vi "Matrix_Transpose.vi"(11 "input matrix":T1) -> (3 "output matrix":T1)   [LabVIEW 2019, in "Trajectory_Library.lvlib"]
doc: "Transpose matrix\n \nInputs:\n - input matrix -- The input matrix\n\nOutputs:\n - output matrix -- The transposed matrix"
uses:
  <vilib>/Analysis/Matrix/Datatypes/RealMatrix.ctl
  Trajectory_Library.lvlib
  <vilib>/Analysis/Matrix/NI_Matrix.lvlib
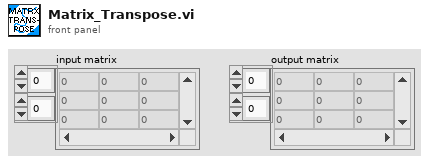
[diagram p1: front panel]
types:
  T1 = typedef "NI_Matrix.lvlib/RealMatrix.ctl" = dbl[][]
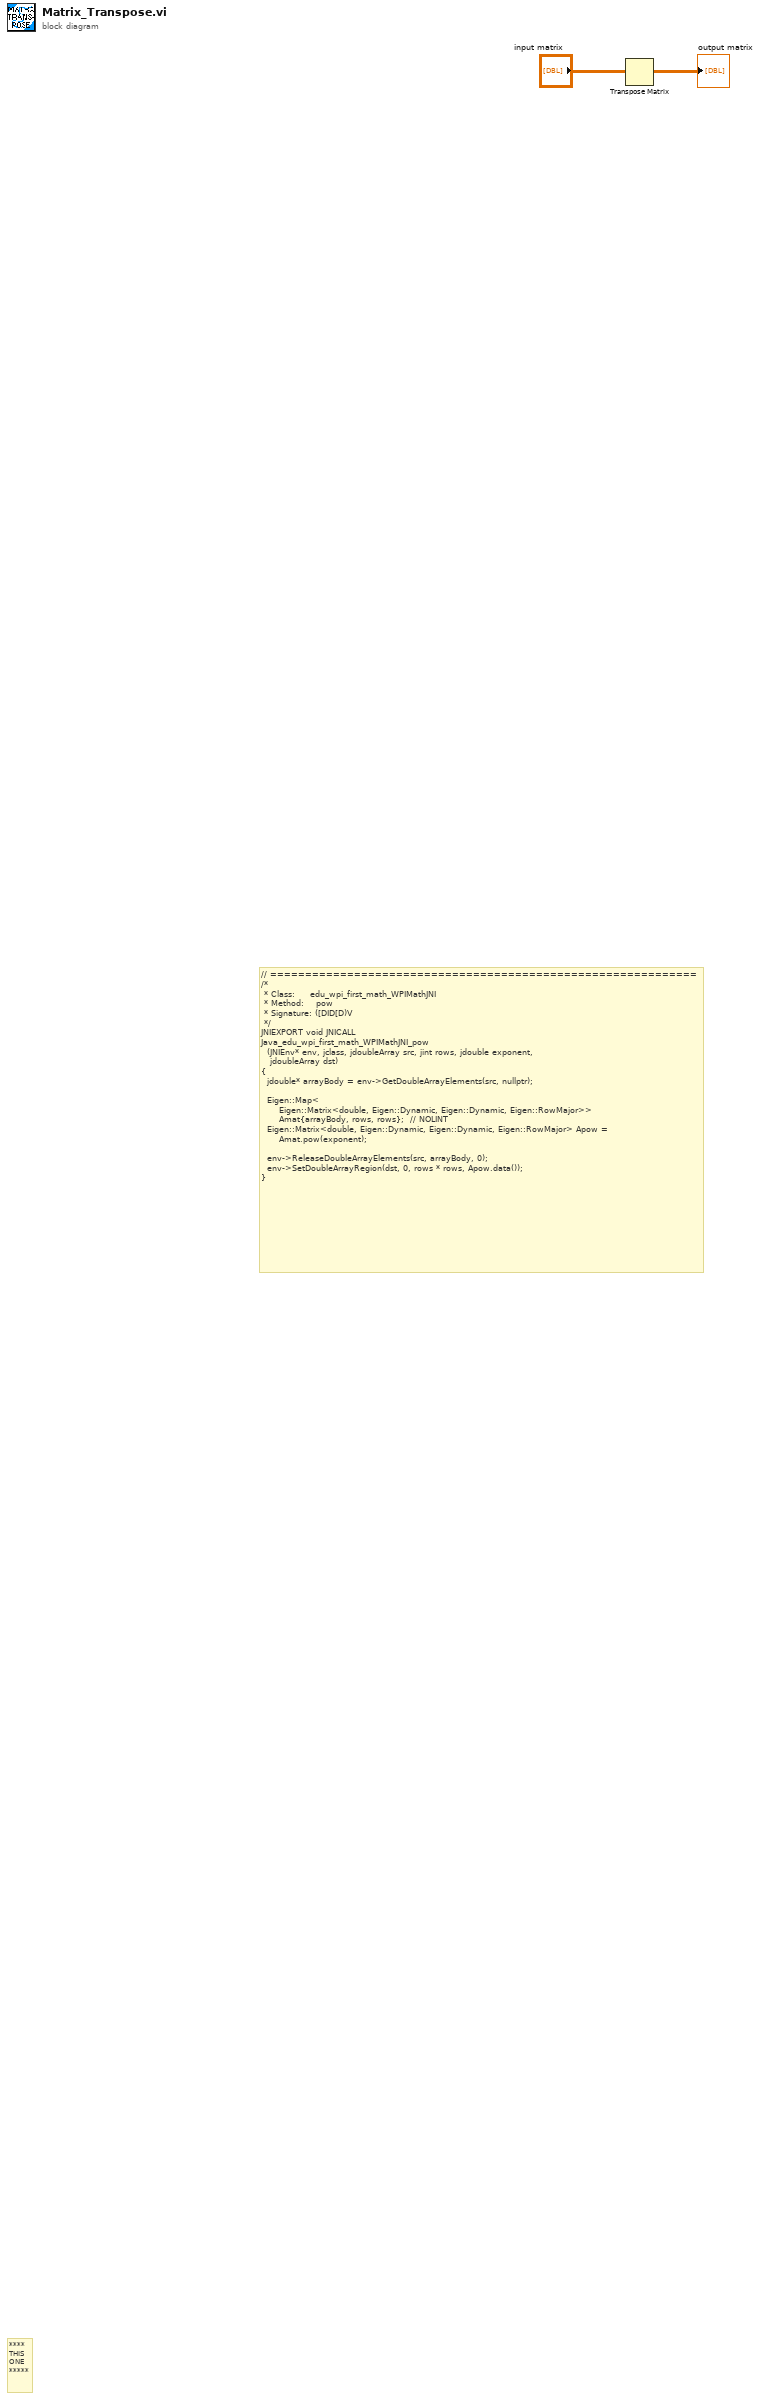
[diagram p0: block diagram]
diagram:
  # "// =============================================================\n/*\n * Class:     edu_wpi_first_math_WPIMathJNI\n * Method:    pow\n * Signature: ([DID[D)V\n */\nJNIEXPORT void JNICALL\nJava_edu_wpi_first_math_WPIMathJNI_pow\n  (JNIEnv* env, jclass, jdoubleArray src, jint rows, jdouble exponent,\n   jdoubleArray dst)\n{\n  jdouble* arrayBody = env->GetDoubleArrayElements(src, nullptr);\n\n  Eigen::Map<\n      Eigen::Matrix<double, Eigen::Dynamic, Eigen::Dynamic, Eigen::RowMajor>>\n      Amat{arrayBody, rows, rows};  // NOLINT\n  Eigen::Matrix<double, Eigen::Dynamic, Eigen::Dynamic, Eigen::RowMajor> Apow =\n      Amat.pow(exponent);\n\n  env->ReleaseDoubleArrayElements(src, arrayBody, 0);\n  env->SetDoubleArrayRegion(dst, 0, rows * rows, Apow.data());\n}"
  # "****\nTHIS\nONE\n*****"
  n1 = Transpose Matrix(1:"input matrix") -> (0:→"output matrix":T1)
